vi "CreateSymbolInDir.vi"(8 "error in":errorcluster, 9 "prefix":string="开发环境", 10 "Name":string="LabVIEW 2014", 11 "Path":path=path "D:/") -> (0 "error out":errorcluster, 3 "Path (dup)":path=path "D:/")   [LabVIEW 2014, in "application.lvclass"]
uses:
  application.lvclass
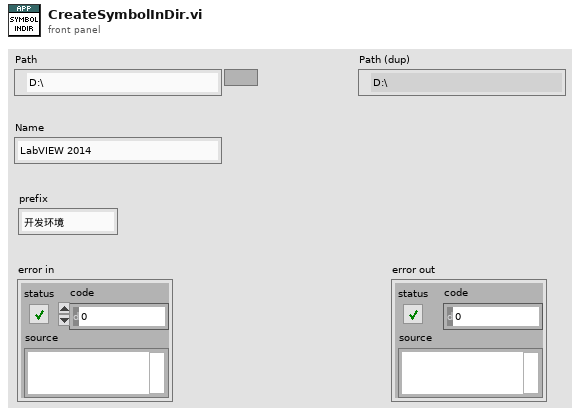
[diagram p1: front panel]
types:
  T1 = enum16{"open", "replace", "create", "open or create", "replace or create", "replace or create with confirmation"}
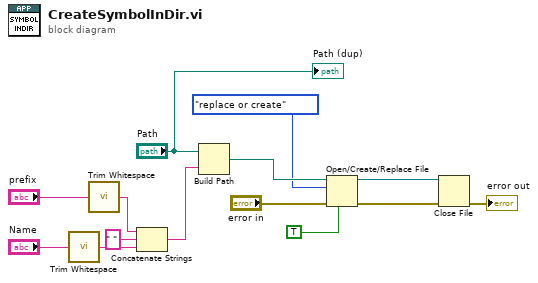
[diagram p0: block diagram]
diagram:
  n1 = call <vilib>:"Trim Whitespace.vi"("string"="Name") -> ("trimmed string"=w3:string)  [unwired: 1 in]
  n2 = call <vilib>:"Trim Whitespace.vi"("string"="prefix") -> ("trimmed string"=w2:string)  [unwired: 1 in]
  n3 = Concatenate Strings(w2, " " ("string"), w3) -> (w6:string)
  n4 = Build Path(base path="Path", name or relative path=w6) -> (appended path=w10:path)
  n5 = Open/Create/Replace File(file path (use dialog)=w10, error in="error in", operation (0:open)=T1."replace or create", disable buffering (F)=TRUE) -> (refnum out=w14:refnum<file>, error out=w13:errorcluster)  [unwired: 2 in, 1 out]
  n6 = Close File(refnum=w14, error in=w13) -> (error out=→"error out":errorcluster)  [unwired: 1 out]
  "Path (dup)" <- "Path"
